vi "OP400ZP_GlobalVariables.vi"() -> ()   [LabVIEW 2020]
uses:
  OP600/SubVI/CheminDeBase.vi
  <vilib>/Utility/config.llb/Read Key (Double).vi
  OP400ZP_VGConf.vi
  <vilib>/Utility/config.llb/Read Key (String).vi
  <vilib>/Utility/config.llb/NI_LVConfig.lvlib
panel:
  out "error out 2":errorcluster caption="error out"
  out "error out":errorcluster
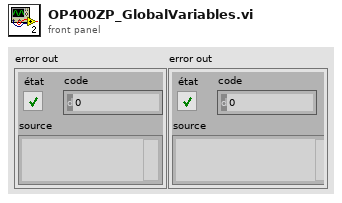
[diagram p1: front panel]
types:
  T1 = typedef "NI_LVConfig.lvlib/Config Data RefNum.ctl" = refnum<k1>
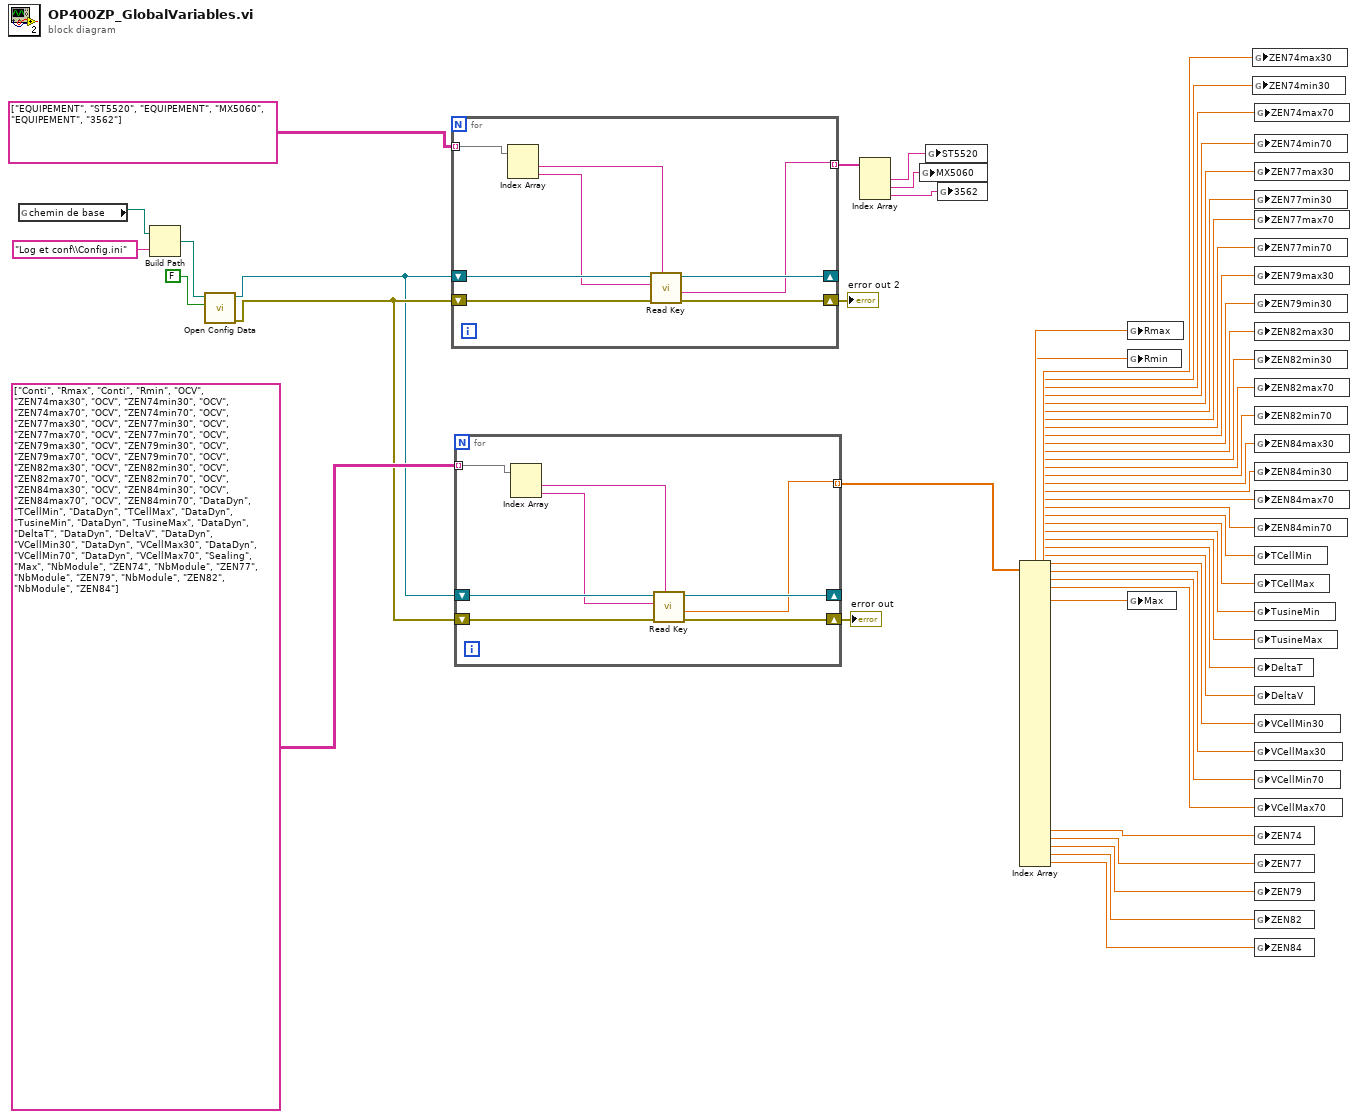
[diagram p0: block diagram]
diagram:
  n1 = global read "CheminDeBase.vi" "chemin de base"() -> (w35:path)
  n2 = Build Path(base path=w35, name or relative path="Log et conf\\Config.ini") -> (appended path=w50:path)
  n3 = call <vilib>:"Open Config Data.vi"("create file if necessary (T)"=FALSE, "configuration file path"=w50) -> ("error out"=w39:errorcluster, "refnum"=w38:T1)  [unwired: 7 in, 1 out]
  n4 = for {
    tunnel: string[][] [["EQUIPEMENT", "ST5520"], ["EQUIPEMENT", "MX5060"], ["EQUIPEMENT", "3562"]] -> [w56] mode=indexing
    shift-right: [w57] -> w36
    shift-left: w39 -> [w59]
    shift-right: [w53] -> _
    shift-left: w38 -> [w58]
    tunnel: [w52] -> w47 mode=indexing
    n5 = Index Array(array=w56) -> (element #1=w55:string, element #2=w54:string)  [unwired: 2 in]
    n6 = call-poly <vilib>:"Read Key.vi"("section"=w55, "error in (no error)"=w59, "key"=w54, "refnum"=w58) -> ("error out"=w57:errorcluster, "value"=w52:string, "refnum out"=w53:T1)  [unwired: 4 in, 1 out]
  }
  "error out 2" <- w36
  n7 = for {
    tunnel: string[][] [["Conti", "Rmax"], ["Conti", "Rmin"], ["OCV", "ZEN74max30"], ["OCV", "ZEN74min30"], ["OCV", "ZEN74max70"], ["OCV", "ZEN74min70"], ["OCV", "ZEN77max30"], ["OCV", "ZEN77min30"], ["OCV", "ZEN77max70"], ["OCV", "ZEN77min70"], ["OCV", "ZEN79max30"], ["OCV", "ZEN79min30"], ["OCV", "ZEN79max70"], ["OCV", "ZEN79min70"], ["OCV", "ZEN82max30"], ["OCV", "ZEN82min30"], ["OCV", "ZEN82max70"], ["OCV", "ZEN82min70"], ["OCV", "ZEN84max30"], ["OCV", "ZEN84min30"], ["OCV", "ZEN84max70"], ["OCV", "ZEN84min70"], ["DataDyn", "TCellMin"], ["DataDyn", "TCellMax"], ["DataDyn", "TusineMin"], ["DataDyn", "TusineMax"], ["DataDyn", "DeltaT"], ["DataDyn", "DeltaV"], ["DataDyn", "VCellMin30"], ["DataDyn", "VCellMax30"], ["DataDyn", "VCellMin70"], ["DataDyn", "VCellMax70"], ["Sealing", "Max"], ["NbModule", "ZEN74"], ["NbModule", "ZEN77"], ["NbModule", "ZEN79"], ["NbModule", "ZEN82"], ["NbModule", "ZEN84"]] -> [w64] mode=indexing
    shift-right: [w65] -> w37
    shift-left: w39 -> [w67]
    shift-right: [w61] -> _
    shift-left: w38 -> [w66]
    tunnel: [w60] -> w42 mode=indexing
    n8 = Index Array(array=w64) -> (element #1=w63:string, element #2=w62:string)  [unwired: 2 in]
    n9 = call-poly <vilib>:"Read Key.vi"("section"=w63, "error in (no error)"=w67, "key"=w62, "refnum"=w66) -> ("error out"=w65:errorcluster, "value"=w60:dbl, "refnum out"=w61:T1)  [unwired: 4 in, 1 out]
  }
  "error out" <- w37
  n10 = Index Array(array=w47) -> (element #1=w46:string, element #2=w45:string, element #3=w44:string)  [unwired: 3 in]
  n11 = global write "OP400ZP_VGConf.vi" "MX5060"(w45) -> ()
  n12 = global write "OP400ZP_VGConf.vi" "ST5520"(w46) -> ()
  n13 = global write "OP400ZP_VGConf.vi" "3562"(w44) -> ()
  n14 = Index Array(array=w42) -> (element #1=w41:dbl, element #2=w40:dbl, element #3=w34:dbl, element #4=w33:dbl, element #5=w32:dbl, element #6=w31:dbl, element #7=w30:dbl, element #8=w29:dbl, element #9=w28:dbl, element #10=w27:dbl, element #11=w26:dbl, element #12=w25:dbl, element #13=w24:dbl, element #14=w23:dbl, element #15=w22:dbl, element #16=w21:dbl, element #17=w20:dbl, element #18=w19:dbl, element #19=w18:dbl, element #20=w17:dbl, element #21=w16:dbl, element #22=w15:dbl, element #23=w14:dbl, element #24=w13:dbl, element #25=w12:dbl, element #26=w11:dbl, element #27=w10:dbl, element #28=w9:dbl, element #29=w8:dbl, element #30=w7:dbl, element #31=w6:dbl, element #32=w5:dbl, element #33=w4:dbl, element #34=w3:dbl, element #35=w2:dbl, element #36=w1:dbl)  [unwired: 36 in]
  n15 = global write "OP400ZP_VGConf.vi" "Rmax"(w41) -> ()
  n16 = global write "OP400ZP_VGConf.vi" "Rmin"(w40) -> ()
  n17 = global write "OP400ZP_VGConf.vi" "Max"(w6) -> ()
  n18 = global write "OP400ZP_VGConf.vi" "ZEN74max30"(w34) -> ()
  n19 = global write "OP400ZP_VGConf.vi" "ZEN74min30"(w33) -> ()
  n20 = global write "OP400ZP_VGConf.vi" "ZEN74max70"(w32) -> ()
  n21 = global write "OP400ZP_VGConf.vi" "ZEN74min70"(w31) -> ()
  n22 = global write "OP400ZP_VGConf.vi" "ZEN77max30"(w30) -> ()
  n23 = global write "OP400ZP_VGConf.vi" "ZEN77min30"(w29) -> ()
  n24 = global write "OP400ZP_VGConf.vi" "ZEN77max70"(w28) -> ()
  n25 = global write "OP400ZP_VGConf.vi" "ZEN77min70"(w27) -> ()
  n26 = global write "OP400ZP_VGConf.vi" "ZEN79max30"(w26) -> ()
  n27 = global write "OP400ZP_VGConf.vi" "ZEN79min30"(w25) -> ()
  n28 = global write "OP400ZP_VGConf.vi" "ZEN82max30"(w24) -> ()
  n29 = global write "OP400ZP_VGConf.vi" "ZEN82min30"(w23) -> ()
  n30 = global write "OP400ZP_VGConf.vi" "ZEN82max70"(w22) -> ()
  n31 = global write "OP400ZP_VGConf.vi" "ZEN82min70"(w21) -> ()
  n32 = global write "OP400ZP_VGConf.vi" "ZEN84max30"(w20) -> ()
  n33 = global write "OP400ZP_VGConf.vi" "ZEN84min30"(w19) -> ()
  n34 = global write "OP400ZP_VGConf.vi" "ZEN84max70"(w18) -> ()
  n35 = global write "OP400ZP_VGConf.vi" "ZEN84min70"(w17) -> ()
  n36 = global write "OP400ZP_VGConf.vi" "TCellMin"(w16) -> ()
  n37 = global write "OP400ZP_VGConf.vi" "TCellMax"(w15) -> ()
  n38 = global write "OP400ZP_VGConf.vi" "TusineMin"(w14) -> ()
  n39 = global write "OP400ZP_VGConf.vi" "TusineMax"(w13) -> ()
  n40 = global write "OP400ZP_VGConf.vi" "DeltaT"(w12) -> ()
  n41 = global write "OP400ZP_VGConf.vi" "DeltaV"(w11) -> ()
  n42 = global write "OP400ZP_VGConf.vi" "VCellMin30"(w10) -> ()
  n43 = global write "OP400ZP_VGConf.vi" "VCellMax30"(w9) -> ()
  n44 = global write "OP400ZP_VGConf.vi" "VCellMin70"(w8) -> ()
  n45 = global write "OP400ZP_VGConf.vi" "VCellMax70"(w7) -> ()
  n46 = global write "OP400ZP_VGConf.vi" "ZEN74"(w5) -> ()
  n47 = global write "OP400ZP_VGConf.vi" "ZEN77"(w4) -> ()
  n48 = global write "OP400ZP_VGConf.vi" "ZEN79"(w3) -> ()
  n49 = global write "OP400ZP_VGConf.vi" "ZEN82"(w2) -> ()
  n50 = global write "OP400ZP_VGConf.vi" "ZEN84"(w1) -> ()
